vi "Restart LabVIEW.vi"(0 "restart?(T)":bool) -> ()   [LabVIEW 2017]
doc: "Restarts LabVIEW when restart?(T) is TRUE. It writes a small restart script, launches it and closes the current instance."
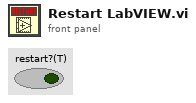
[diagram p1: front panel]
types:
  T1 = enum16{"open", "replace", "create", "open or create", "replace or create", "replace or create with confirmation"}
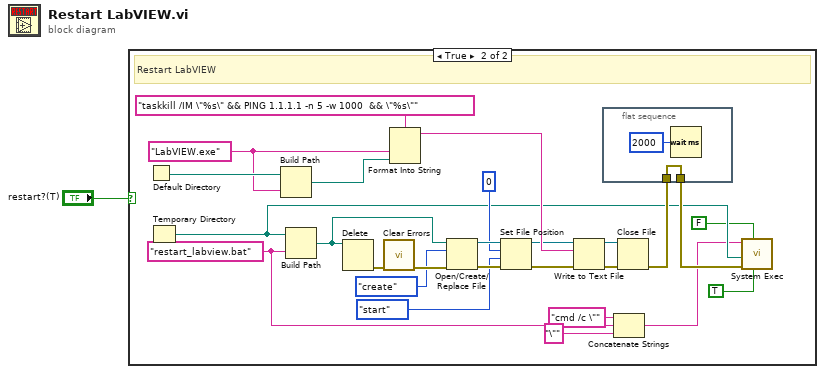
[diagram p0: block diagram]
diagram:
  n1 = case shown="True" "restart?(T)" {
    frame False {
    }
    frame True {
      w8 = "restart_labview.bat"
      w25 = "LabVIEW.exe" ("name or relative path")
      # "Restart LabVIEW"
      n2 = Default Directory() -> (w26:path)
      n3 = Temporary Directory() -> (w7:path)
      n4 = Build Path(base path=w26, name or relative path=w25) -> (appended path=w23:path)
      n5 = Build Path(base path=w7, name or relative path=w8) -> (appended path=w15:path)
      n6 = Delete(path (use dialog)=w15) -> (error out=w24:errorcluster)  [unwired: 4 in, 2 out]
      n7 = call <vilib>:"Clear Errors.vi"("error in (no error)"=w24) -> ("error out"=w16:errorcluster)  [unwired: 5 in, 1 out]
      n8 = Format Into String(format string="taskkill /IM \"%s\" && PING 1.1.1.1 -n 5 -w 1000  && \"%s\"", w25, w23) -> (resulting string=w22:string)  [unwired: 2 in, 1 out]
      n9 = Open/Create/Replace File(file path (use dialog)=w15, error in=w16, operation (0:open)=T1."create") -> (refnum out=w20:refnum<file>, error out=w21:errorcluster)  [unwired: 3 in, 1 out]
      n10 = Set File Position(offset (in bytes) (0)=0, refnum=w20, from (0:start)=enum16{"start", "end", "current"}."start", error in=w21) -> (refnum out=w9:refnum<file>, error out=w17:errorcluster)
      n11 = Write to Text File(file (use dialog)=w9, text=w22, error in=w17) -> (refnum out=w19:refnum<file>, error out=w18:errorcluster)  [unwired: 1 in, 1 out]
      n12 = flat-sequence {
        tunnel: w11 -> [w28]
        tunnel: [w28] -> w10
        frame #0 {
          n13 = Wait (ms)(milliseconds to wait=u32 2000) -> ()  [unwired: 1 out]
        }
      }
      n14 = Concatenate Strings("cmd /c \"" ("string"), w8, "\"" ("string")) -> (w4:string)
      n15 = Close File(refnum=w19, error in=w18) -> (error out=w11:errorcluster)  [unwired: 1 out]
      n16 = call <vilib>:"System Exec.vi"("run minimized? (F)"=TRUE, "wait until completion? (T)"=FALSE, "error in (no error)"=w10, "working directory"=w7, "command line"=w4) -> ()  [unwired: 3 in, 4 out]
    }
  }
